vi "Set DDS Output Gate Enge.vi"(10 "enge":u32, 11 "channel_index":u8) -> ()   [LabVIEW 2021, in "vmmso.lvlib"]
doc: "DLL_API void WINAPI SetDDSOutputGateEnge(unsigned char channel_index, unsigned int enge);"
uses:
  vmmso.lvlib
  vmmso.dll
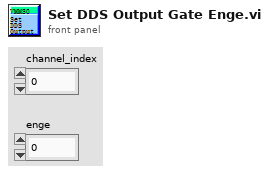
[diagram p1: front panel]
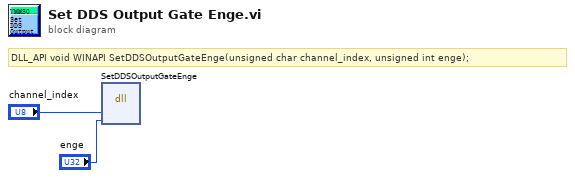
[diagram p0: block diagram]
diagram:
  # "DLL_API void WINAPI SetDDSOutputGateEnge(unsigned char channel_index, unsigned int enge);"
  n1 = dll-call lib="D:/labviewdemo/LabviewDemo 21/vmmso/vmmso.*" fn="SetDDSOutputGateEnge"("channel_index"="channel_index", "enge"="enge") -> ()  [unwired: 6 in, 2 out]
